vi "setEnabledState.vi"(0 "SingleAxisController in":refnum<class "_SingleAxisController.lvclass">, 1 "state (def=DISABLED)":bool, 2 "axes_states (nc - for multi-axis applications only)":T1, 5 "error in (no error)":errorcluster) -> (14 "SingleAxisController out":refnum<class "_SingleAxisController.lvclass">, 17 "success?":bool, 18 "response":string, 19 "error out":errorcluster)   [LabVIEW 2020, in "classes.lvlib" / "_SingleAxisController.lvclass"]
doc: "Produced By:\n\n<B>Kod Integrations, LLC</B>\n4835 Marianne Drive\nMount Airy, MD 21771\nhttp://www.kodintegrations.com\nemail: info@kodintegrations.com\nphone: (240) 687-1288"
uses:
  _SingleAxisController.lvclass
  Controller/_Controller.lvclass
  common/controls/commands.ctl
  libraries/common.lvlib
  C:/GEECS/Developers Version/source/Device Drivers/Newmark-NSC-A/Arcus Driver 3.0.0/ArcusUsbComm/classes/Controller/_Controller.lvclass
  C:/GEECS/Developers Version/source/Device Drivers/Newmark-NSC-A/Arcus Driver 3.0.0/ArcusUsbComm/classes/SingleAxisController/_SingleAxisController.lvclass
  common/controls/motor_enabled_state_axes_group.ctl
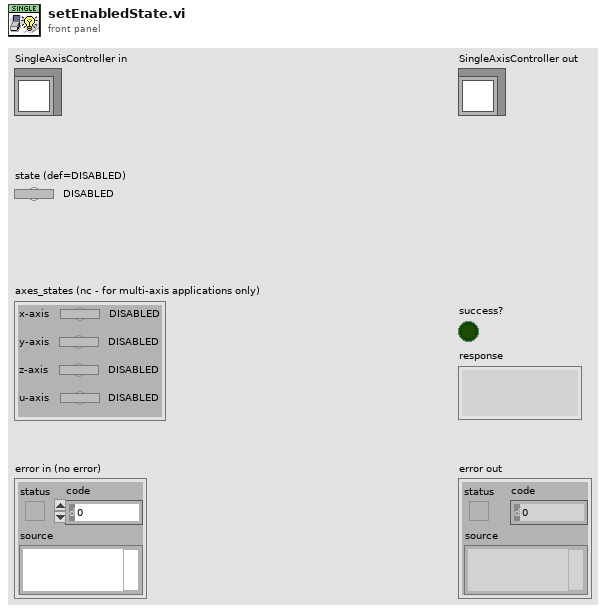
[diagram p1: front panel]
types:
  T1 = typedef "common.lvlib/motor_enabled_state_axes_group.ctl" = cluster{"x-axis":bool, "y-axis":bool, "z-axis":bool, "u-axis":bool}
  T2 = typedef "common.lvlib/commands.ctl" = enum16{"clear error", "constant jog(-)", "constant jog(+)", "get acceleration", "get actual current", "get device name", "get digital input status", "get digital inputs status", "get digital output status", "get digital outputs status", "get firmware ver", "get high speed", "get idle current", "get low speed", "get micro step", "get motor status", "get move mode", "get polarity", "get position", "get product id", "get power status", "get run current", "get status", "home(-)", "home(+)", "move to position", "power down", "power up", "set acceleration", "set device id", "set digital output", "set digital outputs", "set high speed", "set idle current", "set low speed", "set move mode absolute", "set move mode increment", "set polarity", "set position", "set run current", "stop immediate", "stop slow", "store to memory"}
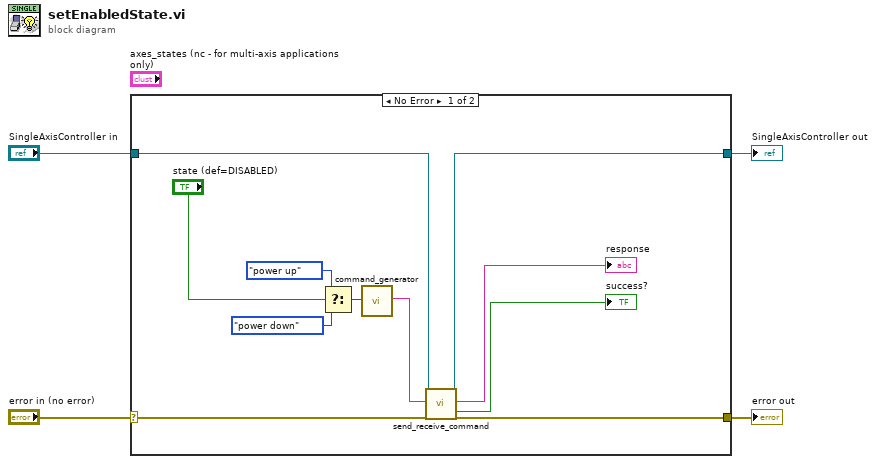
[diagram p0: block diagram]
diagram:
  n1 = case shown="No Error" "error in (no error)" {
    selector: "error in (no error)" -> [w13 w17]
    tunnel: [w12 w17] -> w3
    tunnel: [w10 w16] -> w1
    tunnel: "SingleAxisController in" -> [w11 w16]
    frame No Error {
      n2 = Select(t=commands."power up" ("command"), s="state (def=DISABLED)", f=commands."power down" ("command")) -> (s? t:f=w6:T2)
      n3 = call "command_generator.vi"("cmd (in)"=w6) -> ("ASCII_cmd (out)"=w5:string)  [unwired: 18 in]
      n4 = call "send_receive_command.vi"("reference (in)"=w11, "ASCII Command (in)"=w5, "error in (no error)"=w13) -> ("reference (out)"=w10:refnum<class "_SingleAxisController.lvclass">, "response (out)"=→"response":string, "success?"=→"success?":bool, "error out"=w12:errorcluster)  [unwired: 12 in, 1 out]
    }
    frame Error {
    }
  }
  "error out" <- w3
  "SingleAxisController out" <- w1
